vi "Get UI Details.vi"(8 "error in":errorcluster) -> (0 "error out":errorcluster, 3 "user_interface_details":T1[](array[typedef]))   [LabVIEW 2020, in "MeasurementLink Measurement Server.lvlib"]
uses:
  MeasurementLink Measurement Server.lvlib
  MeasurementLink Measurement Server Internal/RPC Messages/ni_measurementlink_measurement_v1_UserInterfaceDetails.ctl
  Measurement UI.vi
  MeasurementLink Measurement Server Internal/MeasurementLink Measurement Server Internal.lvlib
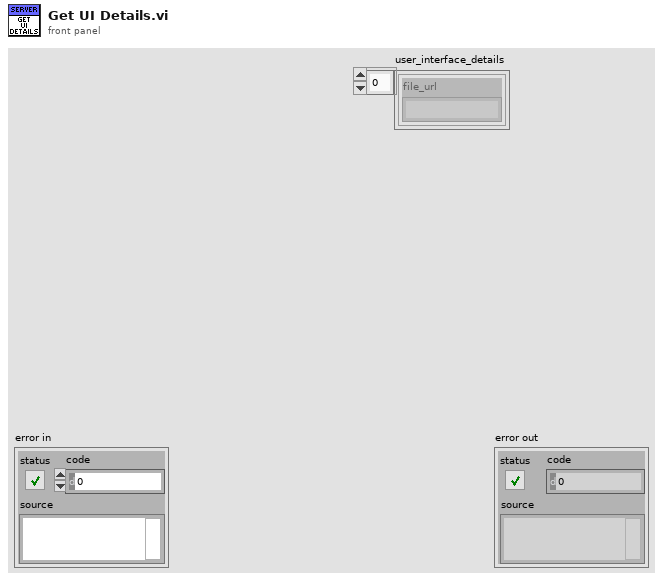
[diagram p1: front panel]
types:
  T1 = typedef "MeasurementLink Measurement Server Internal.lvlib/ni_measurementlink_measurement_v1_UserInterfaceDetails.ctl" = cluster{"file_url":string}
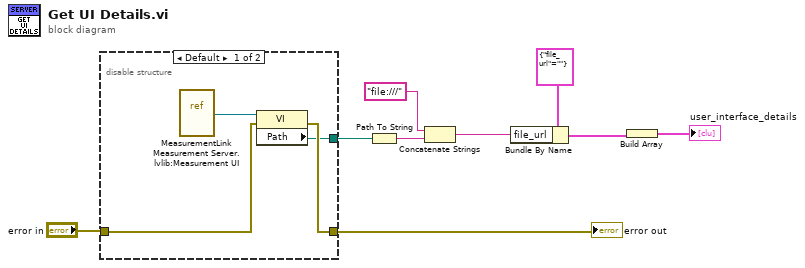
[diagram p0: block diagram]
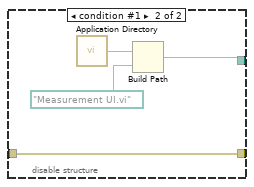
[diagram p2: hidden frame]
diagram:
  n1 = disable-structure shown="Default" {
    disable-tunnel: "error in" -> [w12 w14]
    disable-tunnel: [w11 w14] -> w3
    disable-tunnel: [w10 w15] -> w5
    frame condition #0 (active) {
      n2 = vi-ref "MeasurementLink Measurement Server.lvlib:Measurement UI.vi"() -> (w13:refnum<vi>)
      n3 = property class="VI"(reference=w13, error in=w12) -> (error out=w11:errorcluster, "Path"=w10:path)  [unwired: 1 out]
    }
    frame condition #1 {
      n4 = call <vilib>:"Application Directory.vi"() -> ("Application Directory"=w17:path)
      n5 = Build Path(base path=w17, name or relative path=path "Measurement UI.vi") -> (appended path=w15:path)
    }
  }
  "error out" <- w3
  n6 = Path To String(path=w5) -> (string=w8:string)
  n7 = Concatenate Strings("file:///" ("string"), w8) -> (w7:string)
  n8 = Bundle By Name(cluster=T1 {"file_url"=""} ("UserInterfaceDetails"), "file_url"=w7) -> (w2:T1)
  n9 = Build Array(w2) -> (→"user_interface_details":T1[])
